vi "LED_top.vi"(5 "FPGA I/O In":refnum<k21>="IO Module\\D0 0", 7 "Testpulser On/Off":bool, 8 "State In":enum16{"Initialize", "Get New Value", "Wait"}(ring), 9 "Testpulse Time Delay (20 ns ticks)":u32=15, 10 "Testpulse duration (20 ns ticks)":u32=1, 11 "Address In":u16) -> (0 "Is Test Pulse?":bool)   [LabVIEW 2012]
panel:
  out "Randomly generated testpulse separation input (20 ns ticks)":u32=50000
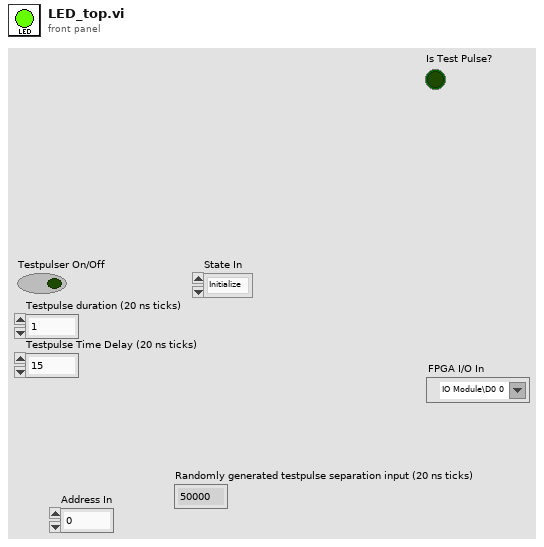
[diagram p1: front panel]
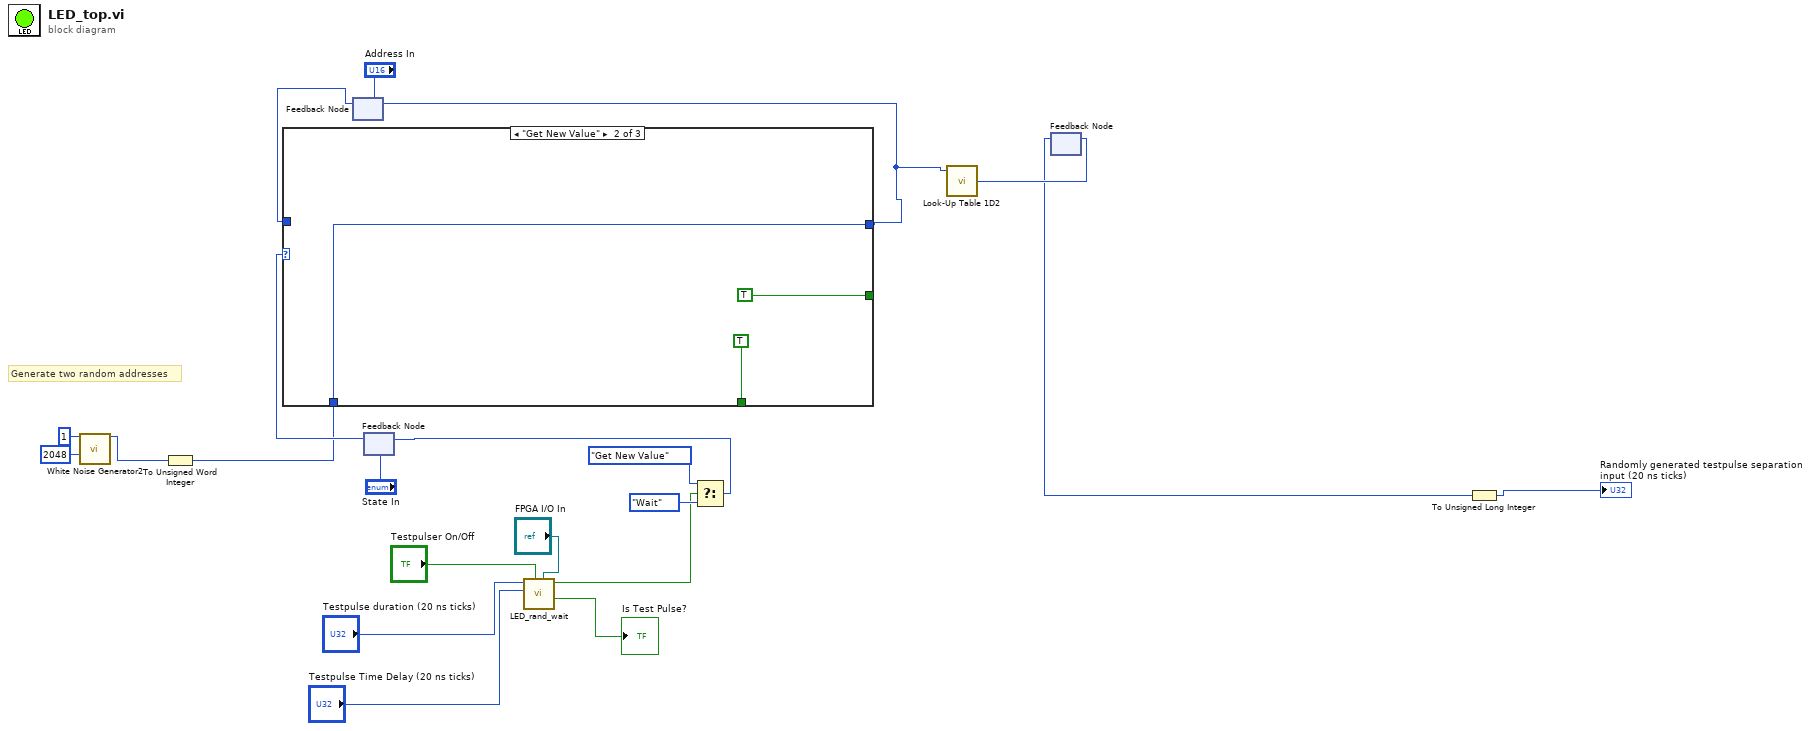
[diagram p0: block diagram]
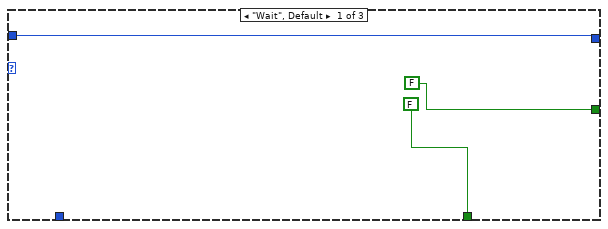
[diagram p2: hidden frame]
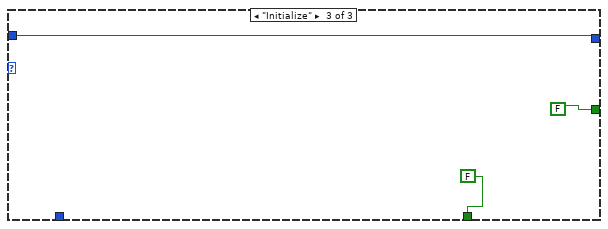
[diagram p3: hidden frame]
diagram:
  # "Generate two random addresses"
  n1 = call "White Noise Generator2"("seed"=u32 1, "amplitude"=u16 2048) -> ("white noise out"=w5:i16)  [unwired: 13 in]
  n2 = To Unsigned Word Integer(number=w5) -> (unsigned 16bit integer=w4:u16)
  n3 = feedback #1("Address In") -> (w11:u16)
  n4 = feedback #2("State In") -> (w17:enum16{"Initialize", "Get New Value", "Wait"})
  n5 = case shown="\"Get New Value\"" w17 {
    tunnel: w11 -> [w22 _ w28]
    tunnel: [FALSE TRUE FALSE] -> _
    tunnel: [FALSE TRUE FALSE] -> _
    tunnel: w4 -> [_ w25 _]
    tunnel: [w22 w25 w28] -> w7
    frame "Wait", Default {
    }
    frame "Get New Value" {
    }
    frame "Initialize" {
    }
  }
  n6 = feedback-in #1(w7) -> ()
  n7 = call "LED_rand_wait.vi"("FPGA I/O In"="FPGA I/O In", "Testpulser On/Off"="Testpulser On/Off", "Testpulse Time Delay (20 ns ticks)"="Testpulse Time Delay (20 ns ticks)", "Testpulse duration (20 ns ticks)"="Testpulse duration (20 ns ticks)") -> ("Is Test Pulse?"=→"Is Test Pulse?":bool, "Get New Value"=w8:bool)  [unwired: 6 in]
  n8 = Select(t=enum16{"Initialize", "Get New Value", "Wait"}."Get New Value", s=w8, f=enum16{"Initialize", "Get New Value", "Wait"}."Wait") -> (s? t:f=w19:enum16{"Initialize", "Get New Value", "Wait"})
  n9 = feedback-in #2(w19) -> ()
  n10 = call "Look-Up Table 1D2"("address"=w7) -> ("data out"=w6:u32)  [unwired: 8 in]
  n11 = feedback #3() -> (w2:u32)  [unwired: 1 in]
  n12 = feedback-in #3(w6) -> ()
  n13 = To Unsigned Long Integer(number=w2) -> (unsigned 32bit integer=→"Randomly generated testpulse separation input (20 ns ticks)":u32)
